vi "Video Processing Target Detection Goes Here.vi"(7 "Update":bool) -> (3 "navX Timestamp":u32)   [LabVIEW 2016]
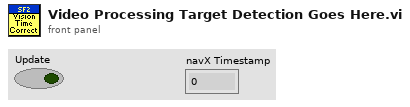
[diagram p1: front panel]
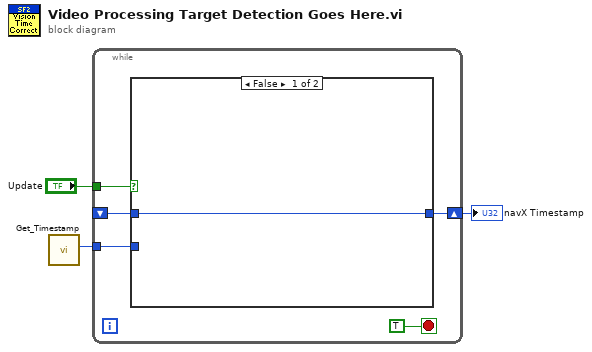
[diagram p0: block diagram]
diagram:
  n1 = call <userlib>:"Get_Timestamp.vi"() -> ("Timestamp"=w2:u32)  [unwired: 11 in]
  n2 = while {
    tunnel: "Update" -> [w7]
    shift-right: [w5] -> w1
    shift-left: _ -> [w4]
    tunnel: w2 -> [w6]
    stop <- TRUE stop-if-true
    n3 = case shown="False" w7 {
      tunnel: w6 -> [_ w10]
      tunnel: [w9 w10] -> w5
      tunnel: w4 -> [w9 _]
      frame False {
      }
      frame True {
      }
    }
  }
  "navX Timestamp" <- w1
